vi "Add Ticket authenticator.vi"(8 "error in (no error)":errorcluster, 9 "Secret":string, 10 "Authentication ID":string, 11 "WAMP Client in":refnum<class "WAMP Client.lvclass">) -> (0 "error out":errorcluster, 3 "WAMP Client out":refnum<class "WAMP Client.lvclass">)   [LabVIEW 2020, in "wamplv.lvlib" / "WAMP Client.lvclass"]
uses:
  WAMP Client.lvclass
  TypeDef/Authentication Method.ctl
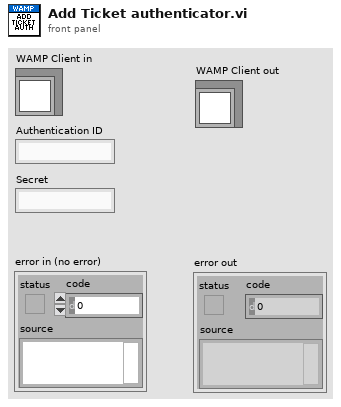
[diagram p1: front panel]
types:
  T1 = typedef "wamplv.lvlib/WAMP Client.lvclass/Authentication Method.ctl" = enum16{"Ticket"}
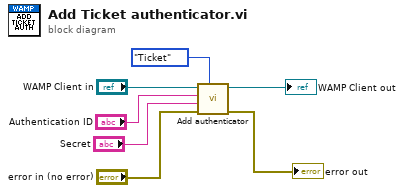
[diagram p0: block diagram]
diagram:
  n1 = call "Add authenticator.vi"("Authentication Method"=Authentication_Method."Ticket", "error in (no error)"="error in (no error)", "Secret"="Secret", "Authentication ID"="Authentication ID", "WAMP Client in"="WAMP Client in") -> ("error out"=→"error out":errorcluster, "WAMP Client out"=→"WAMP Client out":refnum<class "WAMP Client.lvclass">)  [unwired: 5 in]
